vi "Command_logic.vi"(9 "Command Radio Buttons":T2, 10 "Temperature\nto set":dbl) -> (2 "Written command":T1)   [LabVIEW 2022 SP3]
uses:
  Command_buttons.ctl
  Written_command.ctl
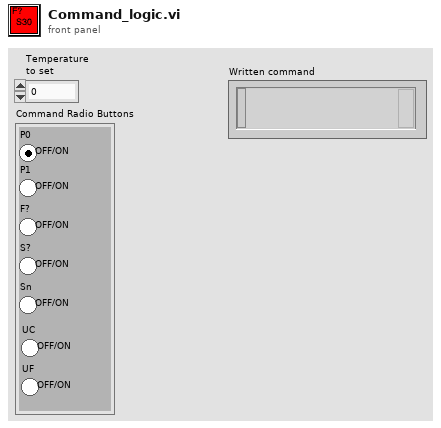
[diagram p1: front panel]
types:
  T1 = typedef "Written_command.ctl" = string
  T2 = typedef "Command_buttons.ctl" = enum32{"P0", "P1", "F?", "S?", "Sn", "UC", "UF"}
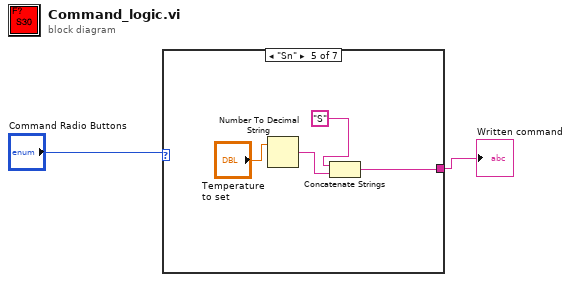
[diagram p0: block diagram]
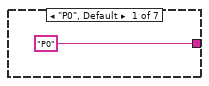
[diagram p2: hidden frame]
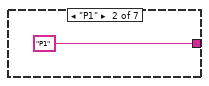
[diagram p3: hidden frame]
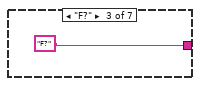
[diagram p4: hidden frame]
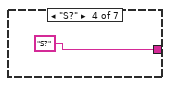
[diagram p5: hidden frame]
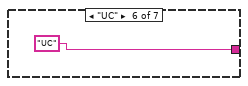
[diagram p6: hidden frame]
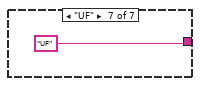
[diagram p7: hidden frame]
diagram:
  n1 = case shown="\"Sn\"" "Command Radio Buttons" {
    tunnel: ["P0" "P1" "F?" "S?" w7 "UC" "UF"] -> w1
    frame "P0", Default {
    }
    frame "P1" {
    }
    frame "F?" {
    }
    frame "S?" {
    }
    frame "Sn" {
      n2 = Number To Decimal String(number="Temperature\nto set") -> (decimal integer string=w9:string)  [unwired: 1 in]
      n3 = Concatenate Strings("S", w9) -> (w7:string)
    }
    frame "UC" {
    }
    frame "UF" {
    }
  }
  "Written command" <- w1
